vi "FF_Bkgnd_correction.vi"(3 "Analogue Data":dbl[][](array[numeric])) -> (0 "Numbers of points":i32[](array[numeric]), 1 "Bkgnd (ppm)":dbl[](array[numeric]))   [LabVIEW 2010]
uses:
  Controls/Multi_run_mode.ctl
  Globals/Meas_global.vi
  Globals/Plug_in_data_global.vi
  Globals/Trav_pos_global.vi
  <vilib>/Analysis/NI_AALBase.lvlib
panel:
  out "Number of Samples":i32
  out "Bkgnd c^2 Values":dbl[](array[numeric])
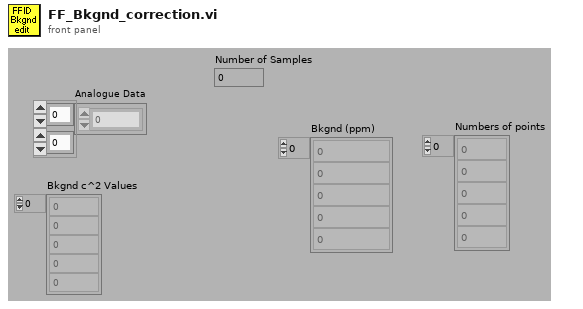
[diagram p1: front panel]
types:
  T1 = typedef "Multi_run_mode.ctl" = enum16{"Move Traverse Only", "Set Tunnel Speed Only", "Set Source Only", "Set Measurement Conditions", "Single Measurement", "Vertical Profile", "Lateral Profile", "Longitudinal Profile", "Explore Volume", "Multi-Axis Profile", "Auto Calibrate", "Meas Fast FID Bkgnd", "Check Beam Power", "Scanning Valve Measurement", "Run VI Named:", "Set ADAM Ch", "Wait (minutes)", "Send Message", "Synchronize With:", "Fall Back to this Row", "Turn Off Row Repeating", "Blank Row"}
  T2 = typedef "Analysis_info_cluster.ctl" = cluster{"Colour":u32, "Inst type":T3, "Inst name":string, "Symbol":string, "Code name":string, "Extra Info":string, "Inst Array":T4, "Index":i32, "Voltage Index":i32, "Extra Titles":string[], "Extra Values":string[]}
  T3 = typedef "Inst_type.ctl" = enum16{"Propeller anemometer", "Raw voltage", "Pressure Transducer", "Pitot-static tube", "Preston tube", "Hot wire", "Cross wire 1", "Cross wire 2", "Generic Linear", "Generic Polynomial", "Generic BackPoly", "Fast FID", "Thermocouple", "Cold wire", "Pulsed Wire", "LDA Vel", "LDA Tran time", "LDA Arr time"}
  T4 = typedef "Instrument_Array.ctl" = enum16{"PWA", "LDA", "Analogue"}
  T5 = typedef "Post_Process.ctl" = enum16{"Take New Data", "Post Process Raw Data File"}
  T6 = typedef "Traverse_cluster.ctl" = cluster{"Start X":dbl, "Start Y":dbl, "Start Z":dbl, "End X":dbl, "End Y":dbl, "End Z":dbl, "No. of pts.":i32, "Spacing":T7, "Filename":path, "Tunnel Speed":dbl, "Averaging time (min)":dbl, "Extra Commands":string, "Specific Arguments":string, "Emission Rate (l/min)":dbl, "Trace Gas Concentration (%)":dbl, "Density Ratio":string, "Comments":string, "Row No":i32, "Row Type Selector":T1, "Completion time":string, "Row Duration (mins)":dbl, "No. of Valid pts.":i32, "Meas Setup File":string}
  T7 = typedef "Spacing.ctl" = enum16{"Linear", "Log", "Gauss", "Specified", "N/A"}
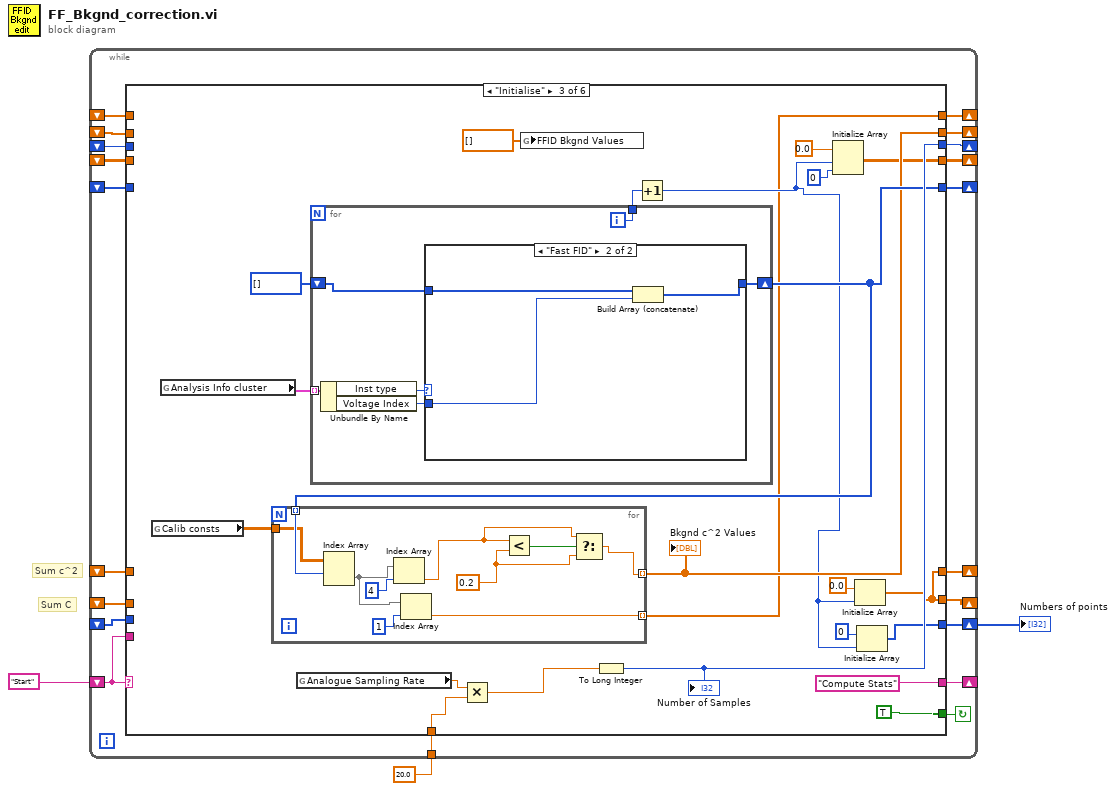
[diagram p0: block diagram]
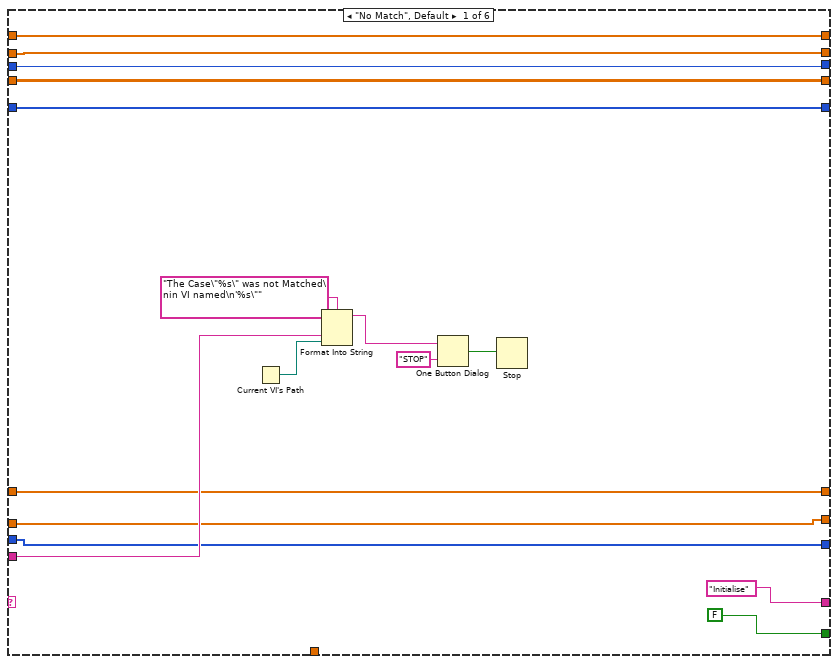
[diagram p2: hidden frame]
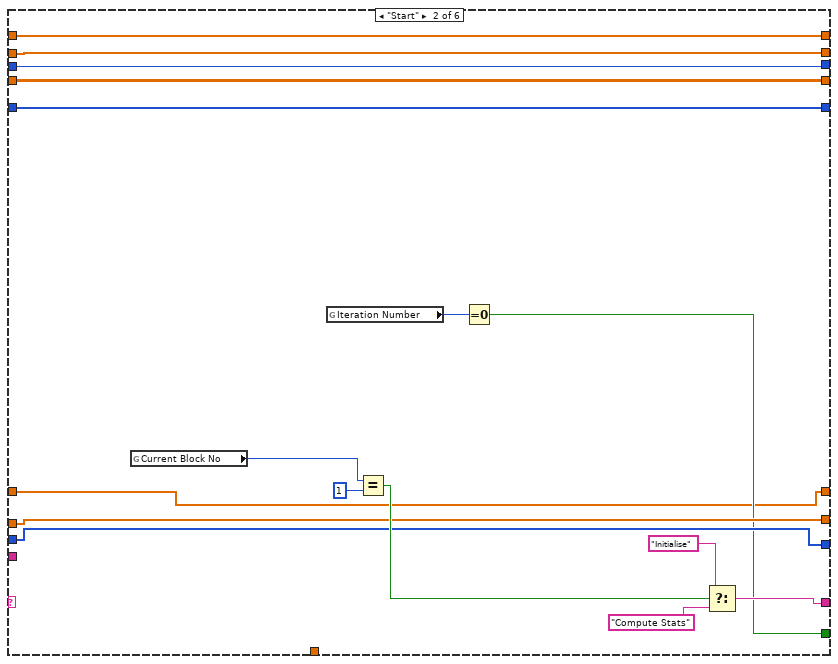
[diagram p3: hidden frame]
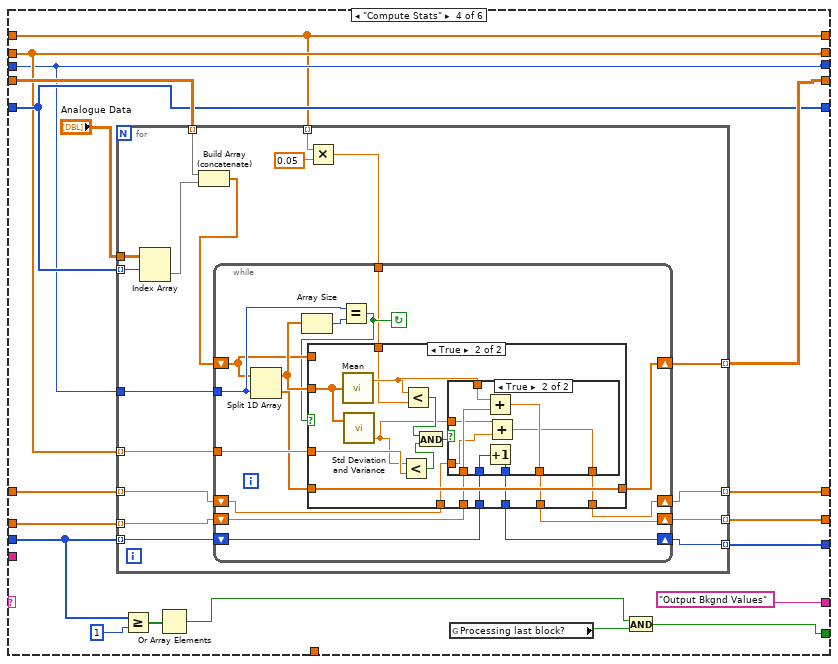
[diagram p5: hidden frame]
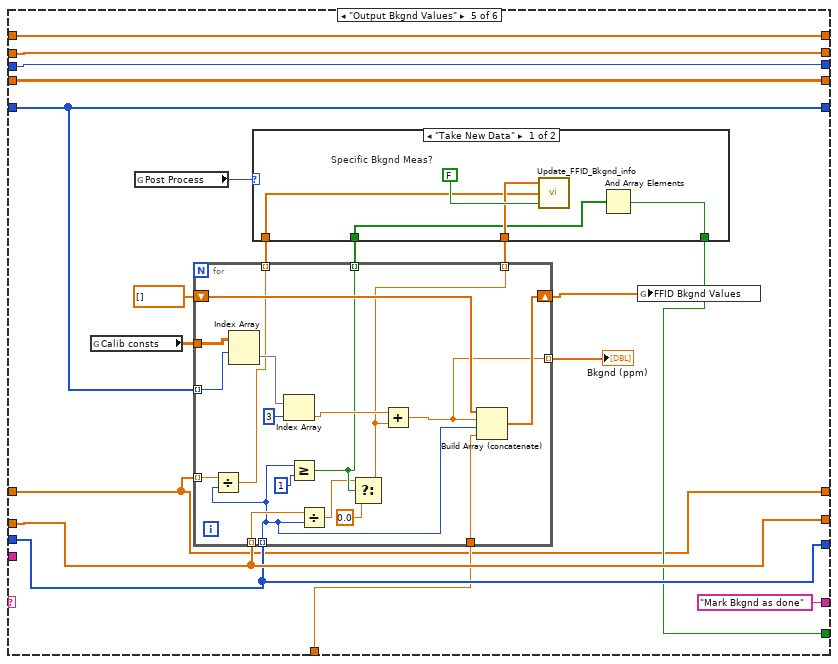
[diagram p8: hidden frame]
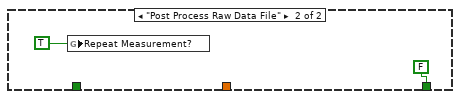
[diagram p9: hidden frame]
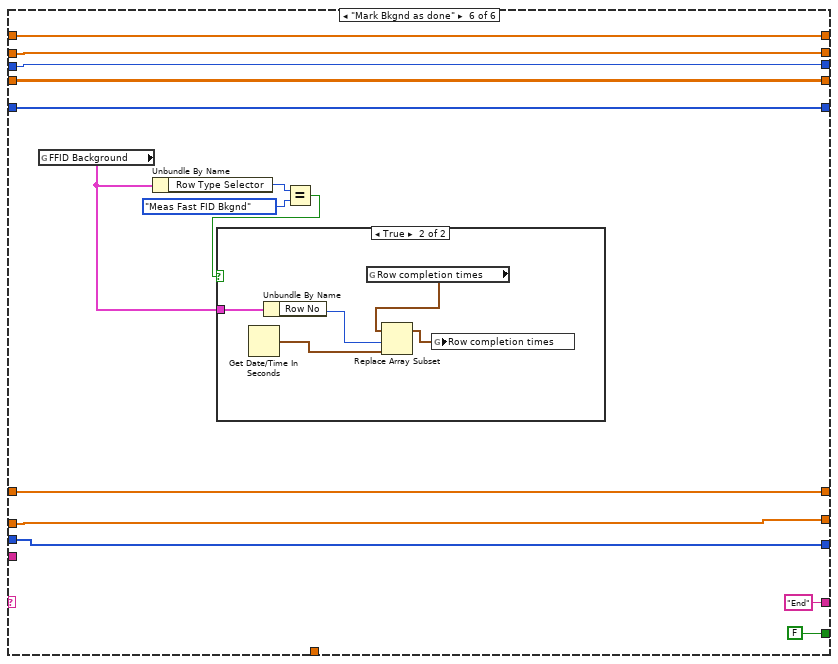
[diagram p10: hidden frame]
diagram:
  # "Sum C"
  # "Sum c^2"
  n1 = while {
    shift-left: "Start" -> [w21]
    shift-right: [w22] -> _
    shift-right: [w20] -> _
    shift-left: _ -> [w18]
    shift-right: [w16] -> _
    shift-left: _ -> [w17]
    shift-right: [w19] -> _
    shift-left: _ -> [w15]
    shift-right: [w14] -> _
    shift-left: _ -> [w13]
    shift-right: [w11] -> _
    shift-left: _ -> [w12]
    shift-right: [w10] -> w2
    shift-left: _ -> [w9]
    tunnel: 20.0 ("y") -> [w8]
    shift-right: [w7] -> _
    shift-left: _ -> [w6]
    shift-right: [w4] -> _
    shift-left: _ -> [w5]
    stop <- w23 continue-if-true
    n2 = case shown="\"Initialise\"" w21 {
      tunnel: [FALSE w42 TRUE w107 w185 FALSE] -> w23
      tunnel: ["Initialise" w52 "Compute Stats" "Output Bkgnd Values" "Mark Bkgnd as done" ("f") "End" ("f")] -> w22
      tunnel: w21 -> [w34 _ _ _ _ _]
      tunnel: [w28 w47 w70 w114 w191 w231] -> w20
      tunnel: [w30 w49 w71 w112 w193 w233] -> w19
      tunnel: w18 -> [w28 w47 _ w114 w191 w231]
      tunnel: w17 -> [w29 w48 _ w116 w192 w232]
      tunnel: [w29 w48 w64 w115 w192 w232] -> w16
      tunnel: w15 -> [w30 w49 _ w112 w193 w233]
      tunnel: [w31 w50 w68 w113 w194 w234] -> w14
      tunnel: w13 -> [w31 w50 _ w113 w194 w234]
      tunnel: w12 -> [w27 w46 _ w111 w197 w236]
      tunnel: [w27 w46 w56 w110 w197 w236] -> w11
      tunnel: [w26 w45 w61 w109 w196 w235] -> w10
      tunnel: w9 -> [w26 w45 _ w105 w196 w235]
      tunnel: w8 -> [_ _ w58 _ w189 _]
      tunnel: [w25 w41 w57 w100 w181 w224] -> w7
      tunnel: w6 -> [w25 w41 _ w100 w181 w224]
      tunnel: w5 -> [w24 w40 _ w99 w180 w223]
      tunnel: [w24 w40 w56 w98 w180 w223] -> w4
      frame "No Match", Default {
        n3 = Current VI's Path() -> (path=w33:path)
        n4 = Format Into String(format string="The Case\"%s\" was not Matched\nin VI named\n'%s\"" ("Format String"), w34, w33) -> (resulting string=w37:string)  [unwired: 2 in, 1 out]
        n5 = One Button Dialog(message=w37, button name ("OK")="STOP") -> (true=w35:bool)
        n6 = Stop(stop? (T)=w35) -> ()
      }
      frame "Start" {
        n7 = global read "Meas_global.vi" "Current Block No"() -> (w44:i32)
        n8 = global read "Meas_global.vi" "Iteration Number"() -> (w43:i32)
        n9 = Equal?(x=w44, y=1) -> (x = y?=w53:bool)
        n10 = Equal To 0?(x=w43) -> (x = 0?=w42:bool)
        n11 = Select(t="Initialise", s=w53, f="Compute Stats") -> (s? t:f=w52:string)
      }
      frame "Initialise" {
        n12 = global read "Meas_global.vi" "Calib consts"() -> (w69:dbl[][])
        n13 = global read "Meas_global.vi" "Analysis Info cluster"() -> (w75:T2[])
        n14 = global read "Meas_global.vi" "Analogue Sampling Rate"() -> (w73:dbl)
        n15 = for {
          tunnel: w75 -> [w93] mode=indexing
          shift-right: [w89] -> w70
          shift-left: i32[] [] -> [w91]
          tunnel: [w88] -> w66
          i -> [w88]
          n16 = Unbundle By Name(w93) -> ("Inst type"=w92:T3, "Voltage Index"=w90:i32)
          n17 = case shown="\"Fast FID\"" w92 {
            tunnel: w91 -> [w94 w97]
            tunnel: w90 -> [_ w96]
            tunnel: [w94 w95] -> w89
            frame "Propeller anemometer", Default {
            }
            frame "Fast FID" {
              n18 = Build Array (concatenate)(w97, w96) -> (w95:i32[])
            }
          }
        }
        n19 = for {
          tunnel: w70 -> [w87] mode=indexing
          tunnel: w69 -> [w86]
          tunnel: [w78] -> w68 mode=indexing
          tunnel: [w82] -> w57 mode=indexing
          w79 = 0.2 ("y")
          n20 = Index Array(array=w86, index (row)=w87) -> (element=w83:dbl[])  [unwired: 1 in]
          n21 = Index Array(array=w83, index=4) -> (element=w80:dbl)
          n22 = Index Array(array=w83, index=1) -> (element=w82:dbl)
          n23 = Less?(x=w80, y=w79) -> (x < y?=w81:bool)
          n24 = Select(t=w80, s=w81, f=w79) -> (s? t:f=w78:dbl)
        }
        "Bkgnd c^2 Values" <- w68
        n25 = Multiply(x=w73, y=w58) -> (x*y=w72:dbl)
        n26 = global write "Plug_in_data_global.vi" "FFID Bkgnd Values"(dbl[] [] ("FFID Bkgnd Values")) -> ()
        n27 = To Long Integer(number=w72) -> (32bit integer=w71:i32)
        "Number of Samples" <- w71
        n28 = Increment(x=w66) -> (x+1=w60:i32)
        n29 = Initialize Array(0.0, w60, 0 ("dimension size")) -> (w64:dbl[][])
        n30 = Initialize Array(0.0, w60) -> (w56:dbl[])
        n31 = Initialize Array(0, w60) -> (w61:i32[])
      }
      frame "Compute Stats" {
        n32 = for {
          tunnel: w114 -> [w133] mode=indexing
          tunnel: "Analogue Data" -> [w132]
          tunnel: w116 -> [w130] mode=indexing
          tunnel: w112 -> [w128]
          tunnel: w113 -> [w127] mode=indexing
          tunnel: [w126] -> w115 mode=indexing
          tunnel: w111 -> [w125] mode=indexing
          tunnel: [w124] -> w110 mode=indexing
          tunnel: w105 -> [w123] mode=indexing
          tunnel: [w122] -> w109 mode=indexing
          tunnel: w100 -> [w120] mode=indexing
          tunnel: w99 -> [w118] mode=indexing
          tunnel: [w117] -> w98 mode=indexing
          n33 = Index Array(array=w132, index (row)=w133) -> (element=w131:dbl[])  [unwired: 1 in]
          n34 = Build Array (concatenate)(w130, w131) -> (w129:dbl[])
          n35 = Multiply(x=w120, y=0.05) -> (x*y=w119:dbl)
          n36 = while {
            shift-right: [w144] -> w126
            shift-left: w129 -> [w143]
            tunnel: w128 -> [w145]
            tunnel: w127 -> [w148]
            shift-right: [w139] -> w124
            shift-left: w125 -> [w140]
            shift-right: [w138] -> w122
            shift-left: w123 -> [w137]
            tunnel: w119 -> [w136]
            shift-right: [w135] -> w117
            shift-left: w118 -> [w134]
            stop <- w141 continue-if-true
            n37 = Split 1D Array(array=w143, index=w145) -> (first subarray=w147:dbl[], second subarray=w142:dbl[])
            n38 = Array Size(array=w147) -> (size(s)=w146:i32)
            n39 = Equal?(x=w145, y=w146) -> (x = y?=w141:bool)
            n40 = case shown="True" w141 {
              tunnel: w148 -> [_ w167]
              tunnel: w147 -> [_ w166]
              tunnel: [w152 w165] -> w144
              tunnel: w143 -> [w152 _]
              tunnel: w142 -> [_ w165]
              tunnel: w140 -> [w151 w164]
              tunnel: [w151 w163] -> w139
              tunnel: [w150 w158] -> w138
              tunnel: w137 -> [w150 w157]
              tunnel: w136 -> [_ w156]
              tunnel: [w149 w155] -> w135
              tunnel: w134 -> [w149 w153]
              frame False {
              }
              frame True {
                n41 = call <vilib>:"Mean.vi"("X"=w166) -> ("mean"=w162:dbl)  [unwired: 1 out]
                n42 = call <vilib>:"Std Deviation and Variance.vi"("X"=w166) -> ("variance"=w154:dbl)  [unwired: 1 in, 2 out]
                n43 = Less?(x=w154, y=w167) -> (x < y?=w160:bool)
                n44 = Less?(x=w162, y=w156) -> (x < y?=w159:bool)
                n45 = And(x=w159, y=w160) -> (x .and. y?=w161:bool)
                n46 = case shown="True" w161 {
                  tunnel: w164 -> [w170 w178]
                  tunnel: [w170 w177] -> w163
                  tunnel: w162 -> [_ w174]
                  tunnel: [w169 w176] -> w158
                  tunnel: w157 -> [w169 w175]
                  tunnel: [w168 w173] -> w155
                  tunnel: w154 -> [_ w172]
                  tunnel: w153 -> [w168 w171]
                  frame False {
                  }
                  frame True {
                    n47 = Add(x=w174, y=w178) -> (x+y=w177:dbl)
                    n48 = Increment(x=w175) -> (x+1=w176:i32)
                    n49 = Add(x=w172, y=w171) -> (x+y=w173:dbl)
                  }
                }
              }
            }
          }
        }
        n50 = Greater Or Equal?(x=w105, y=1) -> (x >= y?=w104:bool[])
        n51 = Or Array Elements(Boolean array=w104) -> (logical OR=w103:bool)
        n52 = global read "Meas_global.vi" "Processing last block?"() -> (w108:bool)
        n53 = And(x=w103, y=w108) -> (x .and. y?=w107:bool)
      }
      frame "Output Bkgnd Values" {
        n54 = global read "Meas_global.vi" "Calib consts"() -> (w195:dbl[][])
        n55 = global read "Meas_global.vi" "Post Process"() -> (w187:T5)
        n56 = for {
          tunnel: w195 -> [w220]
          tunnel: w191 -> [w219] mode=indexing
          tunnel: w197 -> [w217] mode=indexing
          tunnel: w196 -> [w207] mode=indexing
          tunnel: w189 -> [w215]
          shift-right: [w214] -> w186
          shift-left: dbl[] [] -> [w213]
          tunnel: [w211] -> w184 mode=indexing
          tunnel: [w212] -> w183 mode=indexing
          tunnel: [w208] -> w182 mode=indexing
          tunnel: w180 -> [w206] mode=indexing
          tunnel: [w205] -> w179 mode=indexing
          n57 = Divide(x=w206, y=w207) -> (x/y=w205:dbl)
          n58 = Index Array(array=w220, index (row)=w219) -> (element=w218:dbl[])  [unwired: 1 in]
          n59 = Index Array(array=w218, index=3 ("Index")) -> (element=w221:dbl)
          n60 = Greater Or Equal?(x=w207, y=1) -> (x >= y?=w211:bool)
          n61 = Divide(x=w217, y=w207) -> (x/y=w210:dbl)
          n62 = Select(t=w210, s=w211, f=0.0) -> (s? t:f=w208:dbl)
          n63 = Add(x=w221, y=w208) -> (x+y=w212:dbl)
          n64 = Build Array (concatenate)(w213, w212, w207, w215) -> (w214:dbl[])
        }
        "Bkgnd (ppm)" <- w183
        n65 = case shown="\"Take New Data\"" w187 {
          tunnel: w182 -> [w201 _]
          tunnel: [w199 FALSE] -> w185
          tunnel: w184 -> [w200 _]
          tunnel: w179 -> [w198 _]
          frame "Take New Data" {
            w202 = FALSE  # Specific Bkgnd Meas?
            n66 = call "Update_FFID_Bkgnd_info.vi"("Specific Bkgnd Meas?"=w202, "c^2 (ppm^2)"=w198, "C (ppm)"=w201) -> ()  [unwired: 1 in]
            n67 = And Array Elements(Boolean array=w200) -> (logical AND=w199:bool)
          }
          frame "Post Process Raw Data File" {
            n68 = global write "Meas_global.vi" "Repeat Measurement?"(TRUE ("Repeat Measurement?")) -> ()
          }
        }
        n69 = global write "Plug_in_data_global.vi" "FFID Bkgnd Values"(w186) -> ()
      }
      frame "Mark Bkgnd as done" {
        n70 = global read "Trav_pos_global.vi" "FFID Background"() -> (w226:T6)
        n71 = Unbundle By Name(w226) -> ("Row Type Selector"=w228:T1)
        n72 = Equal?(x=w228, y=Multi_run_mode."Meas Fast FID Bkgnd" ("Row Type Selector")) -> (x = y?=w225:bool)
        n73 = case shown="True" w225 {
          tunnel: w226 -> [_ w241]
          frame False {
          }
          frame True {
            n74 = Get Date/Time In Seconds() -> (seconds since 1Jan1904=w237:timestamp)
            n75 = Unbundle By Name(w241) -> ("Row No"=w240:i32)
            n76 = global read "Trav_pos_global.vi" "Row completion times"() -> (w239:timestamp[])
            n77 = Replace Array Subset(array=w239, new element=w237, index=w240) -> (w238:timestamp[])
            n78 = global write "Trav_pos_global.vi" "Row completion times"(w238) -> ()
          }
        }
      }
    }
  }
  "Numbers of points" <- w2
